vi "IntakeExicuteLogic.vi"(9 "HaveAlgae":bool, 11 "HaveCoral":bool) -> (1 "MotorDemandRight":dbl, 2 "MotorDemandLeft":dbl, 3 "MotorDemandTop":dbl, 4 "CurrentState":T1)   [LabVIEW 2023]
uses:
  IntakeStates.ctl
  <vilib>/Rock Robotics/WPI/ThirdParty/JAS_Junk/TrajLib/VI/BoolCmd_Recv_Internal.vi
  <vilib>/Rock Robotics/WPI/ThirdParty/JAS_Junk/TrajLib/VI/DigSeqLogic_Edge_On.vi
  <vilib>/Rock Robotics/WPI/ThirdParty/JAS_Junk/TrajLib/VI/BoolCmd_ObtainQueue.vi
  <vilib>/Rock Robotics/WPI/ThirdParty/JAS_Junk/TrajLib/Trajectory_Library.lvlib
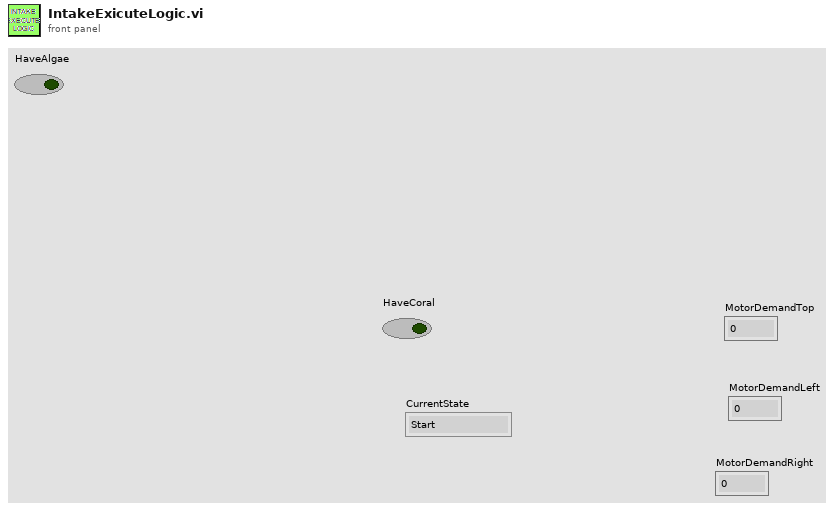
[diagram p1: front panel]
types:
  T1 = typedef "IntakeStates.ctl" = enum16{"Start", "WaitForCommand", "IntakeCoral", "IntakeAlgae", "WaitForCoral", "WaitForAlgae", "DepositCoral", "DepositAlgae", "DepositCoralTimer", "DepositAlgaeTimer"}
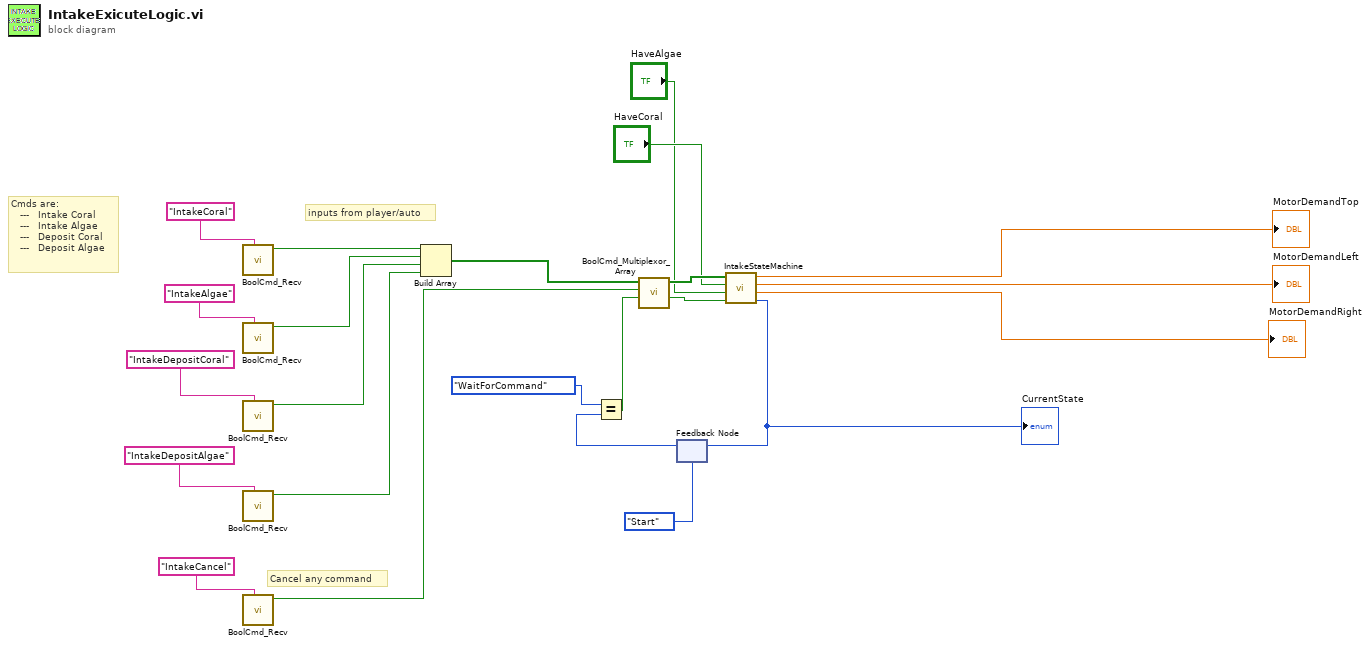
[diagram p0: block diagram]
diagram:
  # "Cmds are:\n   ---   Intake Coral\n   ---   Intake Algae\n   ---   Deposit Coral\n   ---   Deposit Algae"
  # "inputs from player/auto"
  # "Cancel any command"
  n1 = call <vilib>:"BoolCmd_Recv.vi"("Command Name"="IntakeCoral") -> ("New Request"=w18:bool)  [unwired: 9 in, 1 out]
  n2 = call <vilib>:"BoolCmd_Recv.vi"("Command Name"="IntakeAlgae") -> ("New Request"=w17:bool)  [unwired: 9 in, 1 out]
  n3 = call <vilib>:"BoolCmd_Recv.vi"("Command Name"="IntakeDepositCoral") -> ("New Request"=w15:bool)  [unwired: 9 in, 1 out]
  n4 = call <vilib>:"BoolCmd_Recv.vi"("Command Name"="IntakeDepositAlgae") -> ("New Request"=w3:bool)  [unwired: 9 in, 1 out]
  n5 = call <vilib>:"BoolCmd_Recv.vi"("Command Name"="IntakeCancel") -> ("New Request"=w20:bool)  [unwired: 9 in, 1 out]
  n6 = Build Array(w18, w17, w15, w3) -> (w19:bool[])
  n7 = feedback #1(IntakeStates."Start" ("CurrentState")) -> (w10:T1)
  n8 = Equal?(x=IntakeStates."WaitForCommand", y=w10) -> (x = y?=w8:bool)
  n9 = call <vilib>:"BoolCmd_Multiplexor_Array.vi"("Ready"=w8, "Command Cancel"=w20, "Commands"=w19) -> ("Do Cancel"=w13:bool, "Do Command"=w14:bool[])  [unwired: 7 in]
  n10 = call "IntakeStateMachine.vi"("IntakeCancel"=w13, "HaveAlgaeSensor"="HaveAlgae", "HaveCoralSensor"="HaveCoral", "IntakeCommands"=w14) -> ("CurrentState"=w12:T1, "RightMotorDemand"=→"MotorDemandRight":dbl, "LeftMotorDemand"=→"MotorDemandLeft":dbl, "TopMotorDemand"=→"MotorDemandTop":dbl)  [unwired: 4 in]
  "CurrentState" <- w12
  n11 = feedback-in #1(w12) -> ()
